vi "仁科测控通讯.vi"() -> ()   [LabVIEW 2016, in "环境动力监测库.lvlib" / "空调库.lvlib"]
uses:
  <vilib>/Plasmionique/MB Master/MB_Master/MB_Master.lvclass
  <vilib>/Plasmionique/MB Master/MB Master.lvlib
panel:
  out "运行状态":T1
  out "告警状态":T2
  out "传感器状态输出":T3
  out "温湿度解析":cluster{"湿度":dbl, "温度":dbl}
  out "系统参数":u16[](array[numeric])
  out "告警状态":u16[](array[numeric])
  out "传感器状态":u16[](array[numeric])
  out "温湿度解析":u16[](array[numeric])
  in  "读取数据":bool
  in  "释放串口":bool
  in  "打开串口":bool
  out "通讯状态":bool
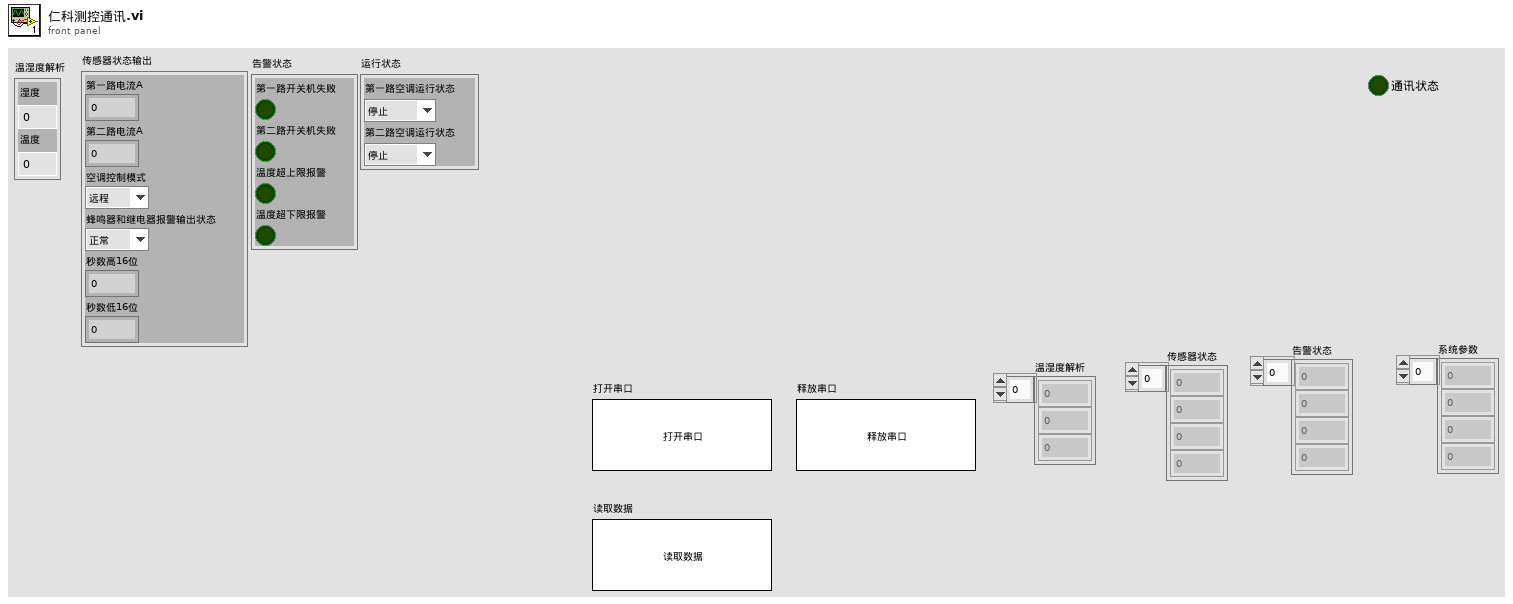
[diagram p1: front panel]
types:
  T1 = cluster{"第一路空调运行状态":enum16{"停止", "制冷", "制热", "未知"}, "第二路空调运行状态":enum16{"停止", "制冷", "制热", "未知"}}
  T2 = cluster{"第一路开关机失败":bool, "第二路开关机失败":bool, "温度超上限报警":bool, "温度超下限报警":bool}
  T3 = cluster{"第一路电流A":u16, "第二路电流A":u16, "空调控制模式":enum16{"远程", "自动"}, "蜂鸣器和继电器报警输出状态":enum16{"正常", "报警"}, "秒数高16位":u16, "秒数低16位":u16}
  T4 = cluster{"型号选择":enum16{"黑盾", "英维克", "仁科测控RS-KTC-N01"}, "MB session in":refnum<class "MB_Master.lvclass">, "英维克空调寄存器":u16[], "通讯状态":bool, "PORT":string, "IP":string, "Slave ID ":u8, "Serial Config":cluster{"baud rate (bps)":u32, "stop bits":u16, "parity":u16, "flow control":u16, "timeout":u32, "retries":i32}, "VISA Resource":refnum<visa-resource-name>, "MB通信方式选择":enum16{"串口", "TCP"}, "系统参数":cluster{"空调开启点":u16, "空调灵敏点":u16, "加热开启点":u16, "加热灵敏度":u16, "高温告警点":u16, "低温告警点":u16}}
  T5 = enum16{"open", "read", "write single", "write", "close"}
  T6 = cluster{"温湿度解析":cluster{"湿度":dbl, "温度":dbl}, "传感器状态输出":cluster{"第一路电流A":u16, "第二路电流A":u16, "空调控制模式":enum16{"远程", "自动"}, "蜂鸣器和继电器报警输出状态":enum16{"正常", "报警"}, "秒数高16位":u16, "秒数低16位":u16}, "告警状态":cluster{"第一路开关机失败":bool, "第二路开关机失败":bool, "温度超上限报警":bool, "温度超下限报警":bool}, "运行状态":cluster{"第一路空调运行状态":enum16{"停止", "制冷", "制热", "未知"}, "第二路空调运行状态":enum16{"停止", "制冷", "制热", "未知"}}}
  T7 = cluster{"第一路电流":u16, "第二路电流":u16, "空调控制模式":enum16{"远程", "自动"}, "蜂鸣器和继电器报警输出状态":enum16{"正常", "报警"}, "秒数高16位":u16, "秒数低16位":u16}
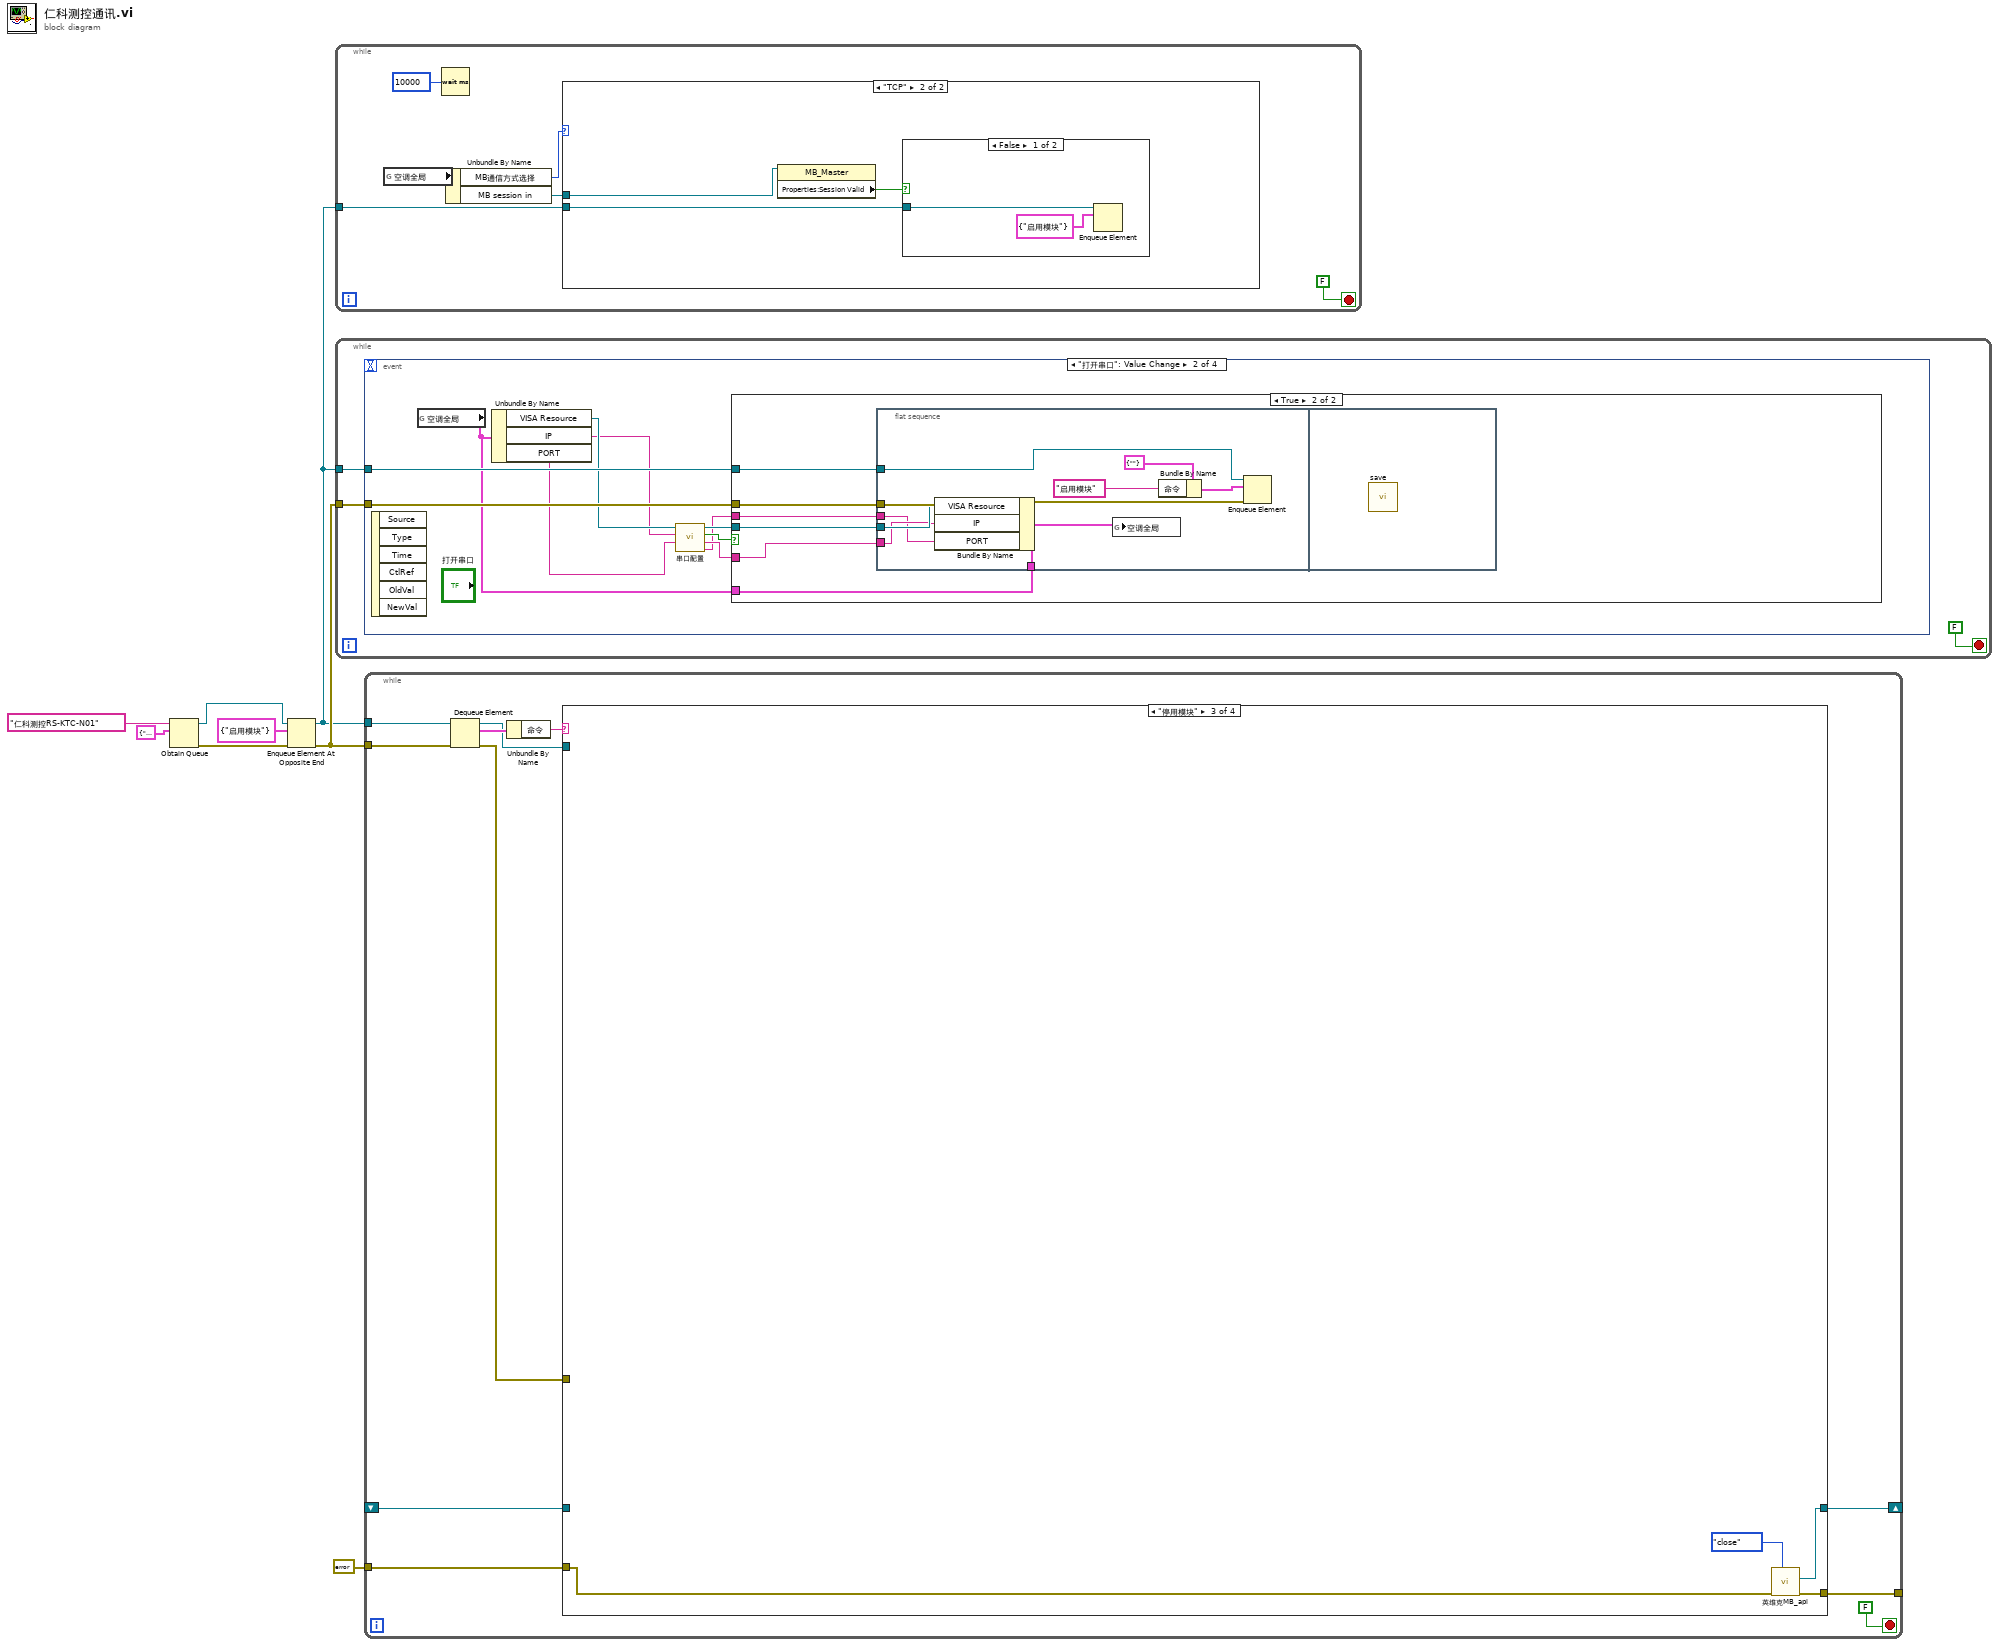
[diagram p0: block diagram]
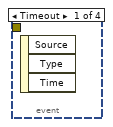
[diagram p4: hidden frame]
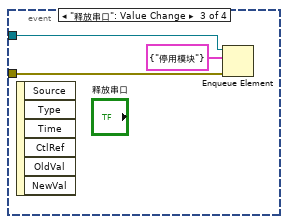
[diagram p6: hidden frame]
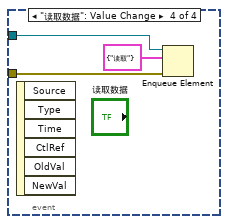
[diagram p7: hidden frame]
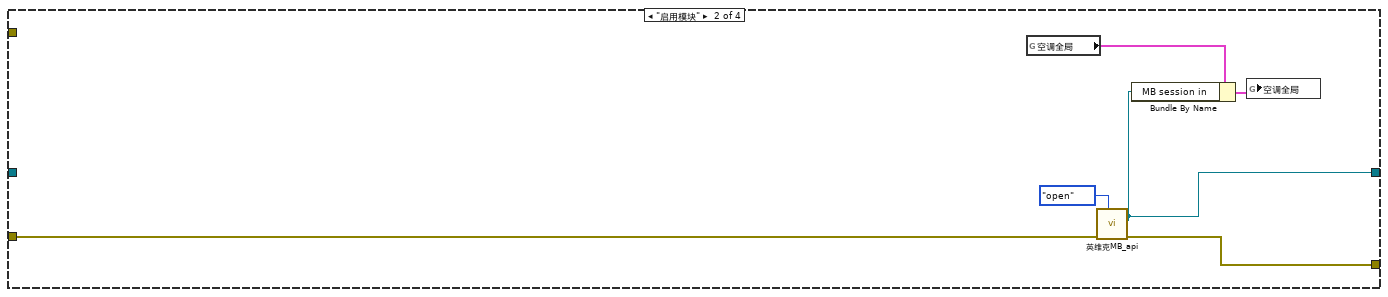
[diagram p9: hidden frame]
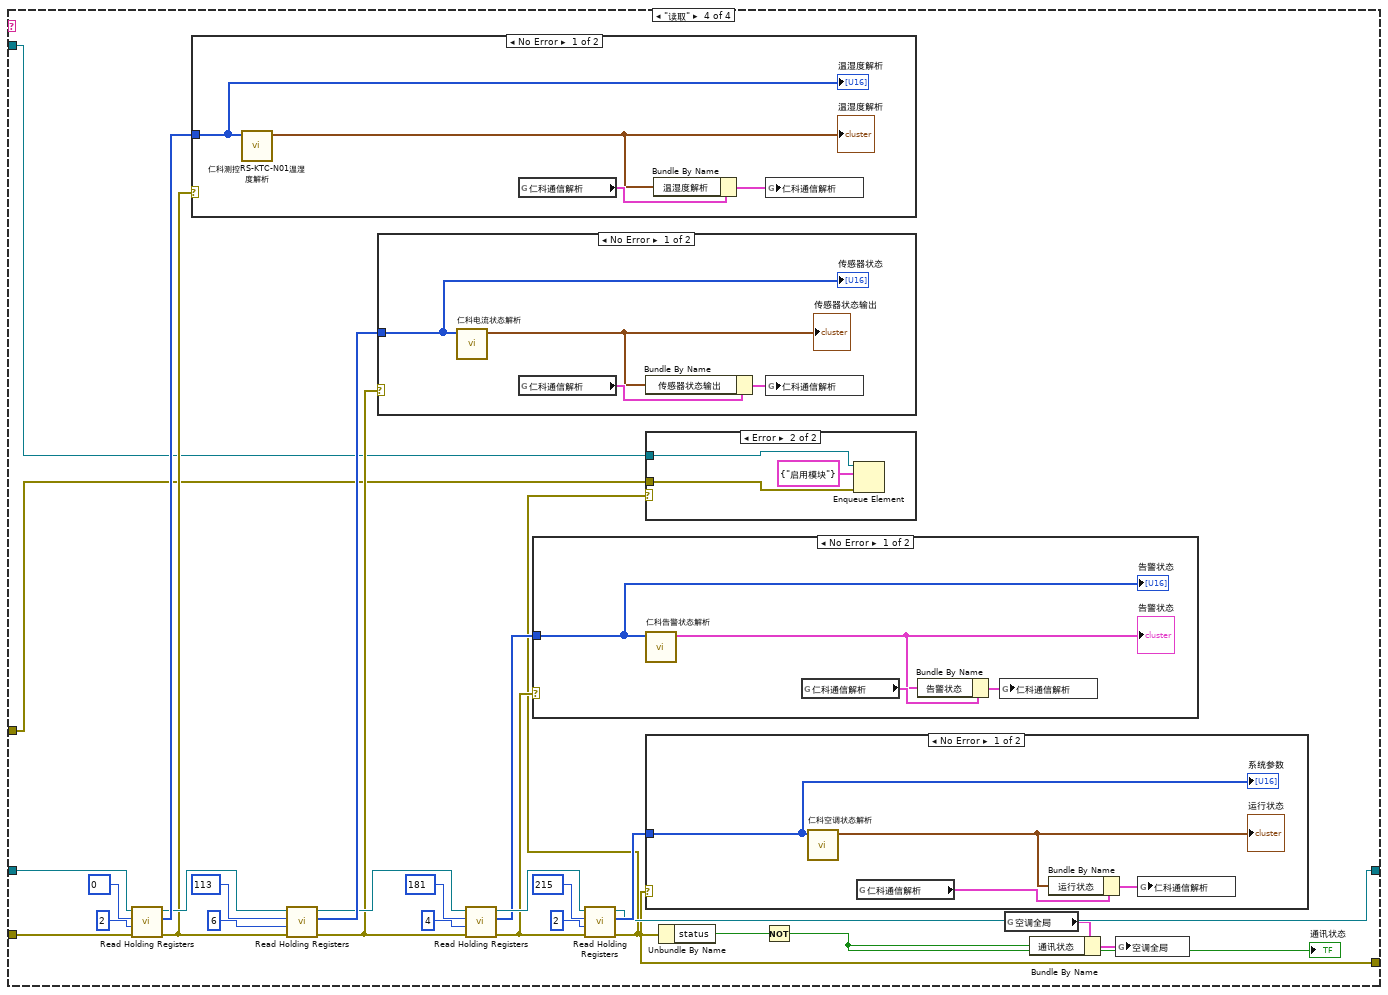
[diagram p10: hidden frame]
diagram:
  n1 = Obtain Queue(name (unnamed)="仁科测控RS-KTC-N01" ("名称（未命名）"), element data type=cluster{"命令":string} {"命令"="启用模块"} ("元素")) -> (queue out=w5:refnum<queue>, error out=w4:errorcluster)  [unwired: 3 in, 1 out]
  n2 = Enqueue Element At Opposite End(queue=w5, element=cluster{"命令":string} {"命令"="启用模块"} ("元素"), error in (no error)=w4) -> (queue out=w1:refnum<queue>, error out=w2:errorcluster)  [unwired: 1 in, 1 out]
  n3 = while {
    tunnel: w1 -> [w14]
    stop <- FALSE stop-if-true
    n4 = global read "断电保存全局变量.vi" "空调全局"() -> (w11:T4)
    n5 = Wait (ms)(milliseconds to wait=u32 10000 ("等待时间（毫秒）")) -> ()  [unwired: 1 out]
    n6 = Unbundle By Name(w11) -> ("MB通信方式选择"=w10:enum16{"串口", "TCP"}, "MB session in"=w9:refnum<class "MB_Master.lvclass">)
    n7 = case shown="\"TCP\"" w10 {
      tunnel: w14 -> [_ w16]
      tunnel: w9 -> [_ w15]
      frame "串口", Default {
      }
      frame "TCP" {
        n8 = property class="MB_Master"(reference=w15) -> ("Properties:Session Valid"=w17:bool)  [unwired: 1 in, 2 out]
        n9 = case shown="False" w17 {
          tunnel: w16 -> [w19 _]
          frame False {
            n10 = Enqueue Element(queue=w19, element=cluster{"命令":string} {"命令"="启用模块"} ("元素")) -> ()  [unwired: 2 in, 3 out]
          }
          frame True {
          }
        }
      }
    }
  }
  n11 = while {
    tunnel: w1 -> [w21]
    tunnel: w2 -> [w20]
    stop <- FALSE stop-if-true
    n12 = event shown="[1] \"打开串口\": Value Change" {
      selector: _ -> [_ _ _ _]
      dyn-events: _ -> [_ _ _ _]
      timeout: _ -> [_ _ _ _]
      tunnel: w21 -> [_ w32 w51 w53]
      tunnel: w20 -> [_ w31 w50 w52]
      event Timeout {
        n13 = event-data() -> ()  [unwired: 1 in, 3 out]
      }
      event "打开串口": Value Change {
        n14 = event-data() -> ()  [unwired: 1 in, 6 out]
        n15 = global read "断电保存全局变量.vi" "空调全局"() -> (w23:T4)
        n16 = Unbundle By Name(w23) -> ("VISA Resource"=w26:refnum<visa-resource-name>, "IP"=w25:string, "PORT"=w24:string)
        n17 = call "串口配置.vi"("PORT"=w24, "IP"=w25, "请选择串口:"=w26) -> ("PORT 2"=w27:string, "IP 2"=w28:string, "确认 2"=w29:bool, "VISA资源名称 2"=w30:refnum<visa-resource-name>)  [unwired: 5 in]
        n18 = case shown="True" w29 {
          tunnel: w30 -> [_ w36]
          tunnel: w32 -> [_ w38]
          tunnel: w31 -> [_ w37]
          tunnel: w28 -> [_ w35]
          tunnel: w27 -> [_ w34]
          tunnel: w23 -> [_ w33]
          frame False {
          }
          frame True {
            n19 = flat-sequence {
              tunnel: w38 -> [w45]
              tunnel: w37 -> [w44]
              tunnel: w36 -> [w41]
              tunnel: w35 -> [w40]
              tunnel: w34 -> [w39]
              tunnel: w33 -> [w43]
              frame #0 {
                n20 = Bundle By Name(cluster=w43, "VISA Resource"=w41, "IP"=w40, "PORT"=w39) -> (w42:T4)
                n21 = global write "断电保存全局变量.vi" "空调全局"(w42) -> ()
                n22 = Bundle By Name(cluster=cluster{"命令":string} {"命令"=""} ("元素"), "命令"="启用模块" ("名称（未命名）")) -> (w46:cluster{"命令":string})
                n23 = Enqueue Element(queue=w45, element=w46, error in (no error)=w44) -> ()  [unwired: 1 in, 3 out]
              }
              frame #1 {
                n24 = call "save.vi"() -> ()  [unwired: 11 in, 1 out]
              }
            }
          }
        }
      }
      event "释放串口": Value Change {
        n25 = event-data() -> ()  [unwired: 1 in, 6 out]
        n26 = Enqueue Element(queue=w51, element=cluster{"命令":string} {"命令"="停用模块"} ("元素"), error in (no error)=w50) -> ()  [unwired: 1 in, 3 out]
      }
      event "读取数据": Value Change {
        n27 = event-data() -> ()  [unwired: 1 in, 6 out]
        n28 = Enqueue Element(queue=w53, element=cluster{"命令":string} {"命令"="读取"} ("元素"), error in (no error)=w52) -> ()  [unwired: 1 in, 3 out]
      }
    }
  }
  n29 = while {
    tunnel: w1 -> [w57]
    tunnel: w2 -> [w64]
    tunnel: [w58] -> _
    shift-right: [w61] -> _
    shift-left: _ -> [w60]
    tunnel: errorcluster {"status"=FALSE, "code"=0, "source"=""} ("error out") -> [w59]
    stop <- FALSE stop-if-true
    n30 = Dequeue Element(queue=w57, error in (no error)=w64) -> (queue out=w56:refnum<queue>, element=w63:cluster{"命令":string}, error out=w55:errorcluster)  [unwired: 1 in, 1 out]
    n31 = Unbundle By Name(w63) -> ("命令"=w62:string)
    n32 = case shown="\"停用模块\"" w62 {
      tunnel: [w67 w69 w75 w82] -> w61
      tunnel: [w66 w73 w76 w81] -> w58
      tunnel: w60 -> [w67 _ _ w105]
      tunnel: w59 -> [w66 w72 w77 w104]
      tunnel: w56 -> [_ _ _ w84]
      tunnel: w55 -> [_ _ _ w83]
      frame Default {
      }
      frame "启用模块" {
        n33 = global read "断电保存全局变量.vi" "空调全局"() -> (w70:T4)
        n34 = call "英维克MB_api.vi"("STEP"=T5."open", "Error in"=w72) -> ("error out"=w73:errorcluster, "MB session out"=w69:refnum<class "MB_Master.lvclass">)  [unwired: 7 in, 1 out]
        n35 = Bundle By Name(cluster=w70, "MB session in"=w69) -> (w68:T4)
        n36 = global write "断电保存全局变量.vi" "空调全局"(w68) -> ()
      }
      frame "停用模块" {
        n37 = call "英维克MB_api.vi"("STEP"=T5."close", "Error in"=w77) -> ("error out"=w76:errorcluster, "MB session out"=w75:refnum<class "MB_Master.lvclass">)  [unwired: 7 in, 1 out]
      }
      frame "读取" {
        n38 = call <vilib>:"Read Holding Registers.vi"("error in (no error)"=w104, "quantity"=u16 2 ("number of holding registers"), "starting address"=u16 0, "MB session in"=w105) -> ("error out"=w101:errorcluster, "Registers"=w103:u16[], "MB session out"=w102:refnum<class "MB_Master.lvclass">)  [unwired: 5 in]
        n39 = case shown="No Error" w101 {
          tunnel: w103 -> [w124 _]
          frame No Error {
            n40 = call "仁科测控RS-KTC-N01温湿度解析.vi"("运行状态输入"=w124) -> ("温湿度解析"=w121:cluster{"湿度":dbl, "温度":dbl})  [unwired: 10 in]
            "温湿度解析" <- w121
            n41 = global read "内部交互全局变量.vi" "仁科通信解析"() -> (w123:T6)
            n42 = Bundle By Name(cluster=w123, "温湿度解析"=w121) -> (w122:T6)
            n43 = global write "内部交互全局变量.vi" "仁科通信解析"(w122) -> ()
            "温湿度解析" <- w124
          }
          frame Error {
          }
        }
        n44 = call <vilib>:"Read Holding Registers.vi"("error in (no error)"=w101, "quantity"=u16 6 ("number of holding registers"), "starting address"=u16 113, "MB session in"=w102) -> ("error out"=w93:errorcluster, "Registers"=w100:u16[], "MB session out"=w94:refnum<class "MB_Master.lvclass">)  [unwired: 5 in]
        n45 = case shown="No Error" w93 {
          tunnel: w100 -> [w120 _]
          frame No Error {
            n46 = call "仁科电流状态解析.vi"("传感器状态输入"=w120) -> ("传感器状态输出"=w117:T7)  [unwired: 10 in]
            "传感器状态输出" <- w117
            n47 = global read "内部交互全局变量.vi" "仁科通信解析"() -> (w119:T6)
            n48 = Bundle By Name(cluster=w119, "传感器状态输出"=w117) -> (w118:T6)
            n49 = global write "内部交互全局变量.vi" "仁科通信解析"(w118) -> ()
            "传感器状态" <- w120
          }
          frame Error {
          }
        }
        n50 = call <vilib>:"Read Holding Registers.vi"("error in (no error)"=w93, "quantity"=u16 4 ("number of holding registers"), "starting address"=u16 181, "MB session in"=w94) -> ("error out"=w87:errorcluster, "Registers"=w86:u16[], "MB session out"=w88:refnum<class "MB_Master.lvclass">)  [unwired: 5 in]
        n51 = case shown="No Error" w87 {
          tunnel: w86 -> [w116 _]
          frame No Error {
            n52 = call "仁科告警状态解析.vi"("告警状态输入"=w116) -> ("告警状态"=w113:T2)  [unwired: 10 in]
            "告警状态" <- w113
            n53 = global read "内部交互全局变量.vi" "仁科通信解析"() -> (w115:T6)
            n54 = Bundle By Name(cluster=w115, "告警状态"=w113) -> (w114:T6)
            n55 = global write "内部交互全局变量.vi" "仁科通信解析"(w114) -> ()
            "告警状态" <- w116
          }
          frame Error {
          }
        }
        n56 = call <vilib>:"Read Holding Registers.vi"("error in (no error)"=w87, "quantity"=u16 2 ("number of holding registers"), "starting address"=u16 215, "MB session in"=w88) -> ("error out"=w81:errorcluster, "Registers"=w85:u16[], "MB session out"=w82:refnum<class "MB_Master.lvclass">)  [unwired: 5 in]
        n57 = case shown="Error" w81 {
          tunnel: w84 -> [_ w108]
          tunnel: w83 -> [_ w106]
          frame No Error {
          }
          frame Error {
            n58 = Enqueue Element(queue=w108, element=cluster{"命令":string} {"命令"="启用模块"} ("元素"), error in (no error)=w106) -> ()  [unwired: 1 in, 3 out]
          }
        }
        n59 = case shown="No Error" w81 {
          tunnel: w85 -> [w112 _]
          frame No Error {
            n60 = call "仁科空调状态解析.vi"("系统参数输入"=w112) -> ("运行状态"=w109:T1)  [unwired: 10 in]
            "运行状态" <- w109
            n61 = global read "内部交互全局变量.vi" "仁科通信解析"() -> (w111:T6)
            n62 = Bundle By Name(cluster=w111, "运行状态"=w109) -> (w110:T6)
            n63 = global write "内部交互全局变量.vi" "仁科通信解析"(w110) -> ()
            "系统参数" <- w112
          }
          frame Error {
          }
        }
        n64 = Unbundle By Name(w81) -> ("status"=w95:bool)
        n65 = Not(x=w95) -> (.not. x?=w78:bool)
        "通讯状态" <- w78
        n66 = global read "断电保存全局变量.vi" "空调全局"() -> (w79:T4)
        n67 = Bundle By Name(cluster=w79, "通讯状态"=w78) -> (w80:T4)
        n68 = global write "断电保存全局变量.vi" "空调全局"(w80) -> ()
      }
    }
  }
